vi "WS1021 Initialize AD7747.vi"(8 "Error In":errorcluster, 11 "FPGA":T1) -> (0 "Error Out":errorcluster)   [LabVIEW 2017]
uses:
  WS_VCAP Driver 039/Source/WSVCAP Shell/Type Defs/WSVCAP SHL FPGA Enum.ctl
  WS_VCAP Driver 039/Source/WSVCAP Shell/Type Defs/WSVCAP SHL I2C DUT Mask Mode Enum.ctl
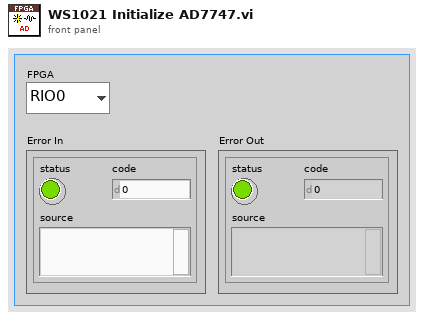
[diagram p1: front panel]
types:
  T1 = typedef "WSVCAP SHL FPGA Enum.ctl" = enum16{"RIO0", "RIO1"}
  T2 = typedef "WSVCAP SHL I2C DUT Mask Mode Enum.ctl" = enum16{"Custom", "All"}
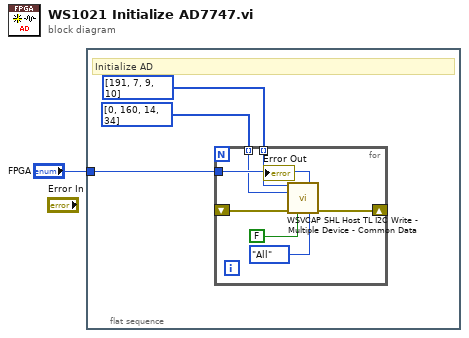
[diagram p0: block diagram]
diagram:
  n1 = flat-sequence {
    tunnel: "FPGA" -> [w4]
    frame #0 {
      # "Initialize AD"
      n2 = for {
        tunnel: w4 -> [w11]
        tunnel: u8[] [191, 7, 9, 10] -> [w10] mode=indexing
        tunnel: u8[] [0, 160, 14, 34] -> [w9] mode=indexing
        shift-right: [w6] -> _
        shift-left: _ -> [w5]
        n3 = call "WSVCAP SHL Host TL I2C Write - Multiple Device - Common Data.vi"("Sub Address"=w10, "FPGA"=w11, "Data Out [U8]"=w9, "error in"=w5, "Log (T)"=FALSE, "DUT Mask Mode (All)"=WSVCAP_SHL_I2C_DUT_Mask_Mode_Enum."All") -> ("error out"=w6:errorcluster)  [unwired: 9 in]
      }
    }
  }
